vi "SetScrollBarVisibility.vi"(0 "reference in":refnum<class "DataGridView.lvclass">, 5 "ScrollBars":i32(ring) items=["None", "Horizontal", "Vertical", "Both"], 11 "error in (no error)":errorcluster) -> (4 "reference out":refnum<class "DataGridView.lvclass">, 15 "error out":errorcluster)   [LabVIEW 2018, in "DataGridView.lvclass"]
doc: "Sets the type of scroll bars to display for the DataGridView control."
uses:
  DataGridView.lvclass
  System.Windows.Forms
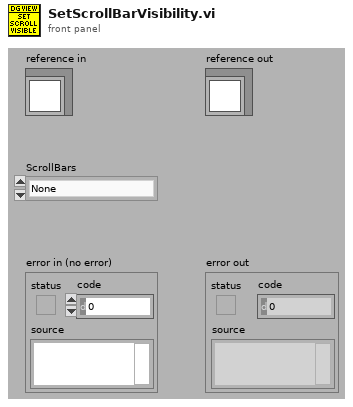
[diagram p1: front panel]
types:
  T1 = typedef "DataGridView.lvclass/ObjectAttributes.ctl" = cluster{"DataGridView":refnum<k24>, "SelectionChangedEvent":refnum<user-event>, "SelectionChanged callback ref":refnum<k27>, "LastSelectedRowIndex":i32}
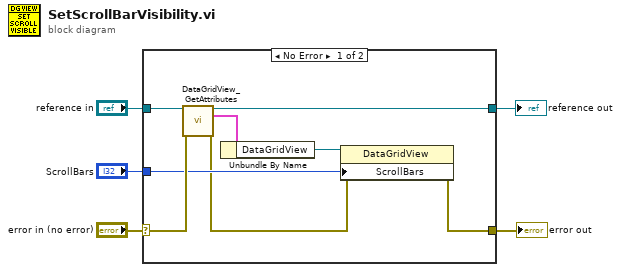
[diagram p0: block diagram]
diagram:
  n1 = case shown="No Error" "error in (no error)" {
    selector: "error in (no error)" -> [w13 w15]
    tunnel: [w6 w15] -> w4
    tunnel: [w10 w14] -> w2
    tunnel: "reference in" -> [w11 w14]
    tunnel: "ScrollBars" -> [w8 _]
    frame No Error {
      n2 = call "DataGridView_GetAttributes.vi"("reference in"=w11, "error in (no error)"=w13) -> ("reference out"=w10:refnum<class "DataGridView.lvclass">, "Data"=w12:T1, "error out"=w7:errorcluster)  [unwired: 10 in, 1 out]
      n3 = Unbundle By Name(w12) -> ("DataGridView"=w9:refnum<k24>)
      n4 = property class="DataGridView"(reference=w9, error in=w7, "ScrollBars"=w8) -> (error out=w6:errorcluster)  [unwired: 1 out]
    }
    frame Error {
    }
  }
  "error out" <- w4
  "reference out" <- w2
